vi "f_create file path.vi"(10 "folder and file name Cluster":T1={"Path"=path "D:/Gantry_General/Main/ms_kao", "folder name"="data", "file name"="data_", "extension"="txt", "add time string"=FALSE}) -> (2 "appended path":path)   [LabVIEW 2016]
panel:
  in  "select / vi path":bool
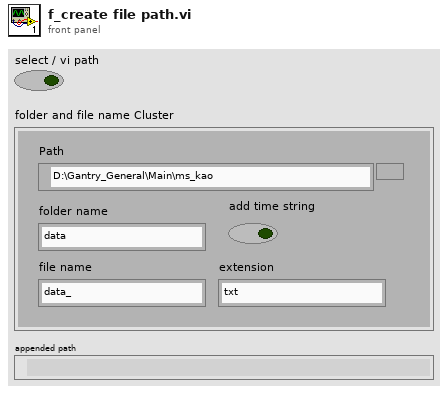
[diagram p1: front panel]
types:
  T1 = cluster{"Path":path, "folder name":string, "file name":string, "extension":string, "add time string":bool}
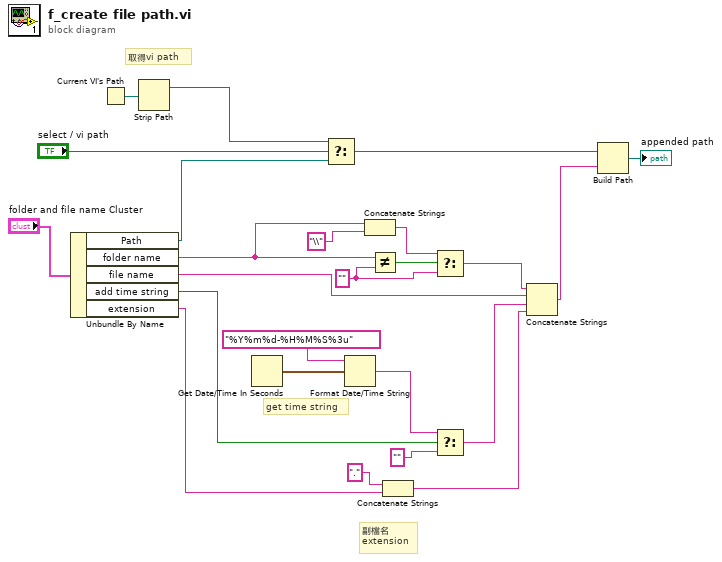
[diagram p0: block diagram]
diagram:
  w11 = ""
  # "副檔名\nextension"
  # "get time string"
  # "取得vi path"
  n1 = Unbundle By Name("folder and file name Cluster") -> ("Path"=w21:path, "folder name"=w17:string, "file name"=w10:string, "add time string"=w6:bool, "extension"=w13:string)
  n2 = Current VI's Path() -> (path=w24:path)
  n3 = Strip Path(path=w24) -> (stripped path=w23:path)  [unwired: 1 out]
  n4 = Get Date/Time In Seconds() -> (seconds since 1Jan1904=w14:timestamp)
  n5 = Select(t=w23, s="select / vi path", f=w21) -> (s? t:f=w20:path)
  n6 = Format Date/Time String(time format string (%c)="%Y%m%d-%H%M%S%3u", seconds (now)=w14) -> (date/time string=w5:string)  [unwired: 1 in]
  n7 = Concatenate Strings(w17, "\\") -> (w16:string)
  n8 = Not Equal?(x=w17, y=w11) -> (x != y?=w18:bool)
  n9 = Concatenate Strings(".", w13) -> (w7:string)
  n10 = Select(t=w16, s=w18, f=w11) -> (s? t:f=w9:string)
  n11 = Select(t=w5, s=w6, f="") -> (s? t:f=w8:string)
  n12 = Concatenate Strings(w9, w10, w8, w7) -> (w3:string)
  n13 = Build Path(base path=w20, name or relative path=w3) -> (appended path=→"appended path":path)
